vi "InitionalizeInstruments.vi"(7 "Address in":refnum<visa-resource-name>, 8 "error in (no error)":errorcluster, 9 "Driver in":path, 10 "Driver 1":path, 11 "VISA Refnum in":refnum<visa-resource-name>) -> (0 "error out":errorcluster, 2 "Instrument out 2":refnum<class "Instrument.lvclass">, 3 "Instrument out":refnum<class "Instrument.lvclass">)   [LabVIEW 2018]
uses:
  Classes/Abstract/Instrument/Instrument/Instrument.lvclass
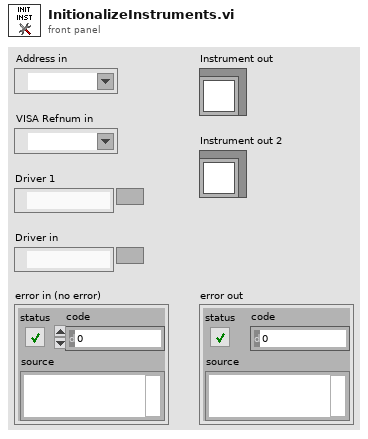
[diagram p1: front panel]
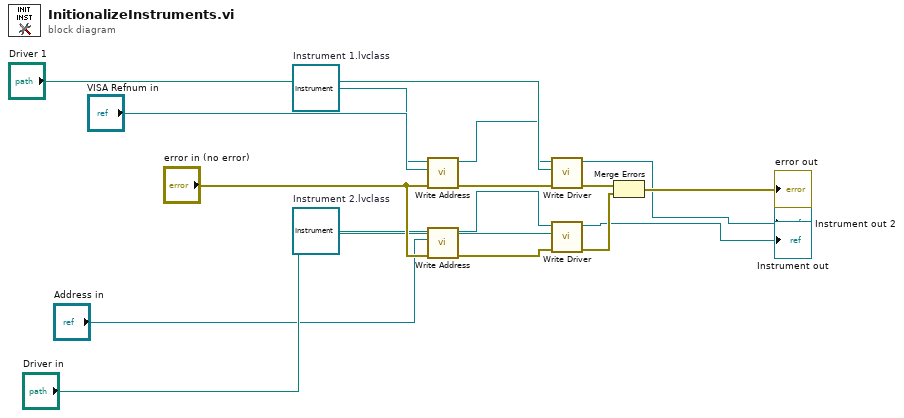
[diagram p0: block diagram]
diagram:
  w3 = refnum<class "Instrument.lvclass"> refnum  # Instrument 2.lvclass
  w1 = refnum<class "Instrument.lvclass"> refnum  # Instrument 1.lvclass
  n1 = call-dynamic "Write Address.vi"("error in (no error)"="error in (no error)", "Address"="VISA Refnum in", "Instrument in"=w1) -> ("error out"=w12:errorcluster, "Instrument out"=w7:refnum<class "Instrument.lvclass">)  [unwired: 7 in]
  n2 = call-dynamic "Write Address.vi"("error in (no error)"="error in (no error)", "Address"="Address in", "Instrument in"=w3) -> ("error out"=w11:errorcluster, "Instrument out"=w5:refnum<class "Instrument.lvclass">)  [unwired: 7 in]
  n3 = call-dynamic "Write Driver.vi"("error in (no error)"=w12, "Driver"="Driver 1", "Instrument in"=w7) -> ("error out"=w13:errorcluster, "Instrument out"=→"Instrument out 2":refnum<class "Instrument.lvclass">)  [unwired: 7 in]
  n4 = call-dynamic "Write Driver.vi"("error in (no error)"=w11, "Driver"="Driver in", "Instrument in"=w5) -> ("error out"=w14:errorcluster, "Instrument out"=→"Instrument out":refnum<class "Instrument.lvclass">)  [unwired: 7 in]
  n5 = Merge Errors(w13, w14) -> (→"error out":errorcluster)
